vi "Main - Search VI Ref.vi"(8 "Error In":errorcluster, 10 "VI Name to Search":string, 11 "VI Refs":refnum<vi>[](array[refnum])) -> (0 "Error Out":errorcluster, 1 "VI Ref Found":refnum<vi>)   [LabVIEW 2020]
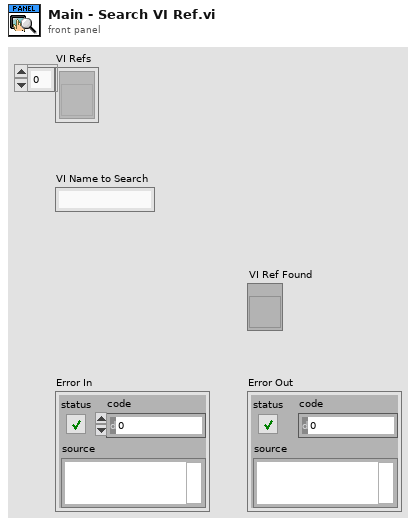
[diagram p1: front panel]
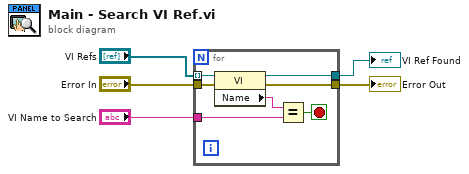
[diagram p0: block diagram]
diagram:
  n1 = for {
    tunnel: "Error In" -> [w12]
    tunnel: [w11] -> w5
    tunnel: "VI Refs" -> [w10] mode=indexing
    tunnel: "VI Name to Search" -> [w8]
    tunnel: [w6] -> w3
    stop <- w7 stop-if-true
    n2 = property class="VI"(reference=w10, error in=w12) -> (reference out=w6:refnum<vi>, error out=w11:errorcluster, "Name"=w9:string)
    n3 = Equal?(x=w9, y=w8) -> (x = y?=w7:bool)
  }
  "Error Out" <- w5
  "VI Ref Found" <- w3
